vi "VI Analyzer Project Provider Wiki.vi"   [LabVIEW 2015]
uses:
  <vilib>/Platform/browser.llb/Open URL in Default Browser (string).vi
panel:
  # "Opening WIKI...."
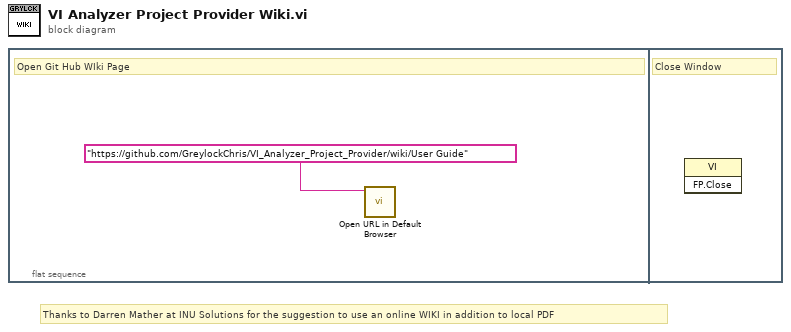
[diagram p0: block diagram]
diagram:
  # "Thanks to Darren Mather at INU Solutions for the suggestion to use an online WIKI in addition to local PDF"
  n1 = flat-sequence {
    frame #0 {
      # "Open Git Hub WIki Page"
      n2 = call-poly <vilib>:"Open URL in Default Browser.vi"("URL"="https://github.com/GreylockChris/VI_Analyzer_Project_Provider/wiki/User Guide") -> ()  [unwired: 5 in, 2 out]
    }
    frame #1 {
      # "Close Window"
      n3 = invoke class="VI" method="FP.Close"() -> ()  [unwired: 3 in, 3 out]
    }
  }
